vi "Test_Calculate Hold-in.vi"(9 "Amps":T1 format="%5.3f A", 10 "Volts":T2 format="%5.3f V", 11 "Table in":refnum<vi>) -> ()   [LabVIEW 2025]
uses:
  Controls/Numeric Voltage.ctl
  Controls/Numeric Current.ctl
panel:
  out "concatenated string":string
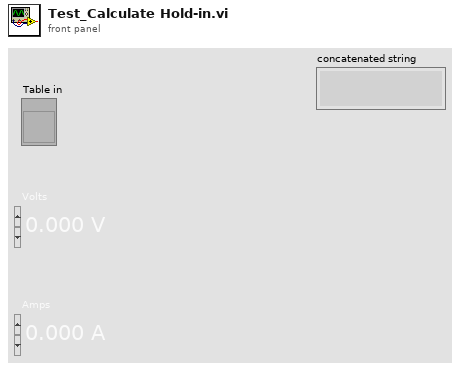
[diagram p1: front panel]
types:
  T1 = typedef "Numeric Current.ctl" = dbl
  T2 = typedef "Numeric Voltage.ctl" = dbl
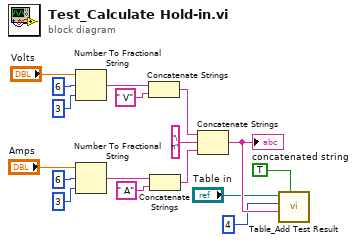
[diagram p0: block diagram]
diagram:
  n1 = Number To Fractional String(number="Volts", width (-)=i16 6, precision (6)=i16 3) -> (F-format string=w13:string)  [unwired: 1 in]
  n2 = Number To Fractional String(number="Amps", width (-)=i16 6, precision (6)=i16 3) -> (F-format string=w10:string)  [unwired: 1 in]
  n3 = Concatenate Strings(w13, " V" ("string")) -> (w9:string)
  n4 = Concatenate Strings(w10, " A" ("string")) -> (w8:string)
  n5 = Concatenate Strings(w9, "\n" ("string"), w8) -> (w6:string)
  "concatenated string" <- w6
  n6 = call "Table_Add Test Result.vi"("Pass?"=TRUE, "Test Result"=w6, "index (row)"=4, "Table in"="Table in") -> ()  [unwired: 7 in, 1 out]
